vi "Close.vi"(8 "error in":errorcluster, 11 "IModulate Voltage in":refnum<class "IModulate Voltage.lvclass">) -> (0 "error out":errorcluster, 3 "IModulate Voltage out":refnum<class "IModulate Voltage.lvclass">)   [LabVIEW 2023, in "IModulate Voltage.lvclass"]
uses:
  IModulate Voltage.lvclass
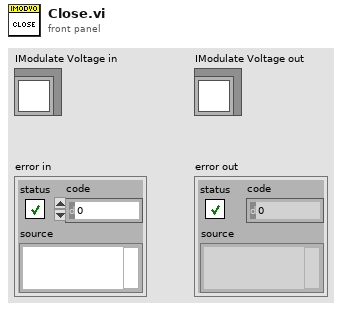
[diagram p1: front panel]
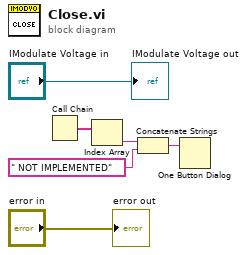
[diagram p0: block diagram]
diagram:
  n1 = Call Chain() -> (call chain=w4:string[])
  n2 = Index Array(array=w4) -> (element=w1:string)  [unwired: 1 in]
  n3 = Concatenate Strings(w1, " NOT IMPLEMENTED" ("string")) -> (w3:string)
  n4 = One Button Dialog(message=w3) -> ()  [unwired: 1 in, 1 out]
  "error out" <- "error in"
  "IModulate Voltage out" <- "IModulate Voltage in"
